vi "Returning Values By Reference Array Of Simple Struct.vi"(8 "error in (no error)":errorcluster, 10 "length":i32, 11 "circleArray":i32) -> (0 "error out":errorcluster, 3 "circleArray out":i32)   [LabVIEW 2009, in "LabVIEWWrapper_PassingDataSampleDLL.lvlib"]
doc: "void ReturningValuesByReference_ArrayOfSimpleStruct (struct simpleStructCircle **circleArray, int length);"
uses:
  LabVIEWWrapper_PassingDataSampleDLL.lvlib
  PassingDataSampleDLL.dll
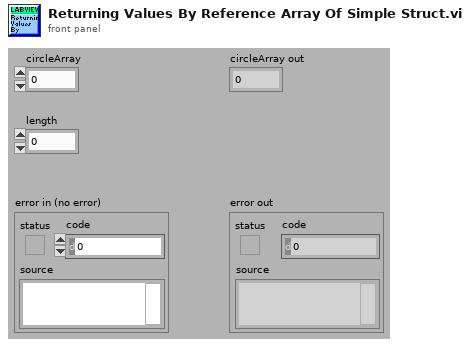
[diagram p1: front panel]
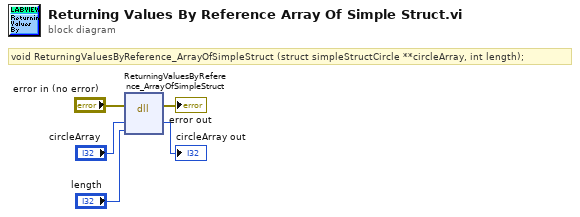
[diagram p0: block diagram]
diagram:
  # "void ReturningValuesByReference_ArrayOfSimpleStruct (struct simpleStructCircle **circleArray, int length);"
  n1 = dll-call lib="C:/My Dropbox/Systems Engineering Application/SDK/C Integration/LabVIEWWrapper/PassingDataSampleDLL.*" fn="ReturningValuesByReference_ArrayOfSimpleStruct"(error in="error in (no error)", "circleArray"="circleArray", "length"="length") -> (error out=→"error out":errorcluster, "circleArray"=→"circleArray out":i32)  [unwired: 4 in, 1 out]
